vi "readData.vi"(8 "error in (no error)":errorcluster, 10 "Header":T1, 11 "M1M3SAL in":refnum<class "M1M3SAL.lvclass">) -> (0 "error out":errorcluster, 2 "Data":variant, 3 "M1M3SAL out":refnum<class "M1M3SAL.lvclass">)   [LabVIEW 2016, in "M1M3SupportCommunicator.lvlib" / "M1M3SAL.lvclass"]
uses:
  M1M3SAL.lvclass
  DataTypes/MessageHeader.ctl
  DataTypes/MessageTypes.ctl
  DataTypes/MessageTopics.ctl
  Common_RT_Utilities/U8ArrayParserAutoIndexing/U8ArrayParserAutoIndexing.lvclass
  M1M3SupportCommunicator.lvlib
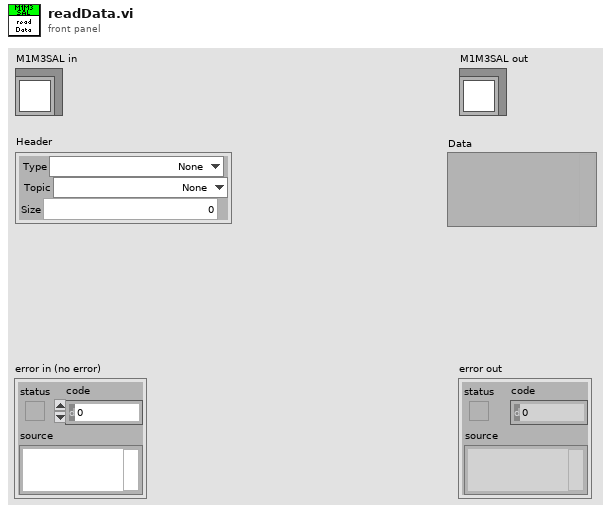
[diagram p1: front panel]
types:
  T1 = typedef "M1M3SupportCommunicator.lvlib/MessageHeader.ctl" = cluster{"Type":T2, "Topic":T3, "Size":i32}
  T2 = typedef "M1M3SupportCommunicator.lvlib/MessageTypes.ctl" = enum8{"None", "PutSample", "GetNextSample", "LogEvent", "GetEvent", "IssueCommand", "CommandId", "WaitForCompletion", "AcceptCommand", "AckCommand"}
  T3 = typedef "M1M3SupportCommunicator.lvlib/MessageTopics.ctl" = enum8{"None", "ForceActuatorData", "MirrorForceData", "HardpointData", "AirData", "DynamicData", "FPGAData", "IMSData", "ForceActuatorStatus", "ElevationData", "HardpointStatus", "HardpointActuatorChase", "AirStatus", "ForceActuatorSafetyChecks", "ForceActuatorTest", "ActuatorBroadcastCounter", "StatusChecks", "CellChecks", "HardpointActuatorBreakaway", "RaiseMirrorComplete", "ILCCommunication", "ElevationAngleChecks", "DetailedState", "ServoLoops", "ForceActuatorInfo", "LowerMirrorComplete", "HardpointActuatorInfo", "SettingsApplied", "ErrorCode", "StartupChecks", "SummaryState", "SettingVersions", "ActuatorTestStatus", "AppliedSettingsMatchStart", "Enable", "EnterMaintenance", "Standby", "AbortLowerM1M3", "ApplyAberrationByForces", "ApplyAOSCorrectionByBendingModes", "ClearAOSCorrection", "Start", "RaiseM1M3", "TestForceActuator", "LowerM1M3", "ApplyAOSCorrectionByForces", "Disable", "ApplyAberationByBendingMode", "TestHardpoint", "ManipulateM1M3", "ClearAberration", "Exit", "TestAir", "AbortRaiseM1M3", "MoveHardpointActuators", "ExitMaintenance", "Shutdown"}
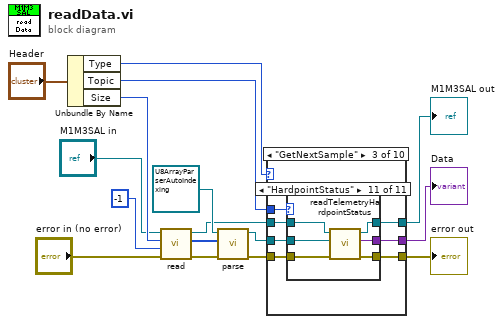
[diagram p0: block diagram]
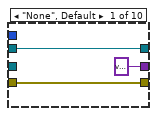
[diagram p2: hidden frame]
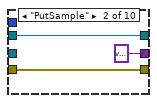
[diagram p3: hidden frame]
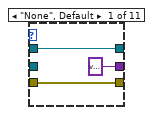
[diagram p4: hidden frame]
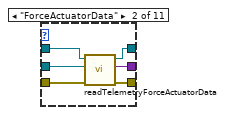
[diagram p5: hidden frame]
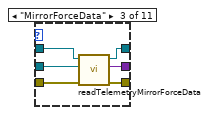
[diagram p6: hidden frame]
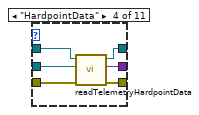
[diagram p7: hidden frame]
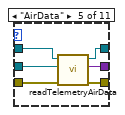
[diagram p8: hidden frame]
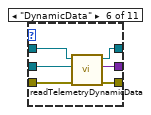
[diagram p9: hidden frame]
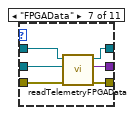
[diagram p10: hidden frame]
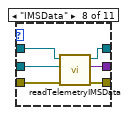
[diagram p11: hidden frame]
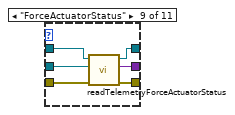
[diagram p12: hidden frame]
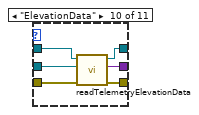
[diagram p13: hidden frame]
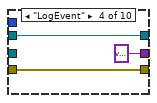
[diagram p14: hidden frame]
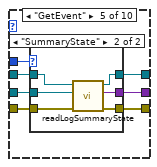
[diagram p15: hidden frame]
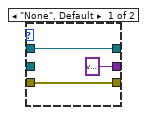
[diagram p16: hidden frame]
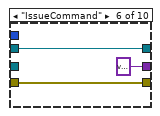
[diagram p17: hidden frame]
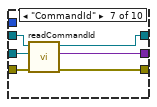
[diagram p18: hidden frame]
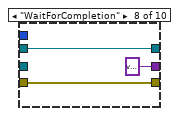
[diagram p19: hidden frame]
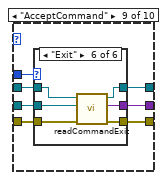
[diagram p20: hidden frame]
diagram:
  n1 = Unbundle By Name("Header") -> ("Type"=w1:T2, "Topic"=w15:T3, "Size"=w14:i32)
  n2 = call "read.vi"("error in (no error)"="error in (no error)", "Timeout"=-1, "NumberOfBytes"=w14, "M1M3SAL in"="M1M3SAL in") -> ("error out"=w6:errorcluster, "Data"=w10:u8[], "M1M3SAL out"=w9:refnum<class "M1M3SAL.lvclass">)  [unwired: 4 in, 1 out]
  n3 = call "parse.vi"("error in (no error)"=w6, "Data"=w10, "U8ArrayParserAutoIndexing in"=refnum<class "U8ArrayParserAutoIndexing.lvclass"> refnum ("RTUtilities.lvlib:U8ArrayParserAutoIndexing.lvclass")) -> ("error out"=w7:errorcluster, "U8ArrayParserAutoIndexing out"=w8:refnum<class "U8ArrayParserAutoIndexing.lvclass">)  [unwired: 7 in]
  n4 = case shown="\"GetNextSample\"" w1 {
    tunnel: w15 -> [_ _ w29 _ w96 _ _ _ w130 _]
    tunnel: w9 -> [w19 w22 w27 w95 w102 w114 w119 w123 w129 w166]
    tunnel: w8 -> [_ _ w23 _ w101 _ w118 _ w128 _]
    tunnel: w7 -> [w17 w21 w25 w93 w100 w113 w117 w121 w127 w164]
    tunnel: [w19 w22 w28 w95 w97 w114 w116 w123 w126 w166] -> w4
    tunnel: [variant ("EventSummaryState") variant ("EventSummaryState") w24 variant ("EventSummaryState") w98 variant ("EventSummaryState") w120 variant ("EventSummaryState") w125 variant ("EventSummaryState")] -> w3
    tunnel: [w17 w21 w26 w93 w99 w113 w115 w121 w124 w164] -> w2
    frame "None", Default {
    }
    frame "PutSample" {
    }
    frame "GetNextSample" {
      n5 = case shown="\"HardpointStatus\"" w29 {
        tunnel: [w32 w33 w43 w49 w55 w61 w67 w73 w79 w85 w91] -> w28
        tunnel: w27 -> [w32 w38 w44 w50 w56 w62 w68 w74 w80 w86 w92]
        tunnel: [w31 w35 w40 w46 w53 w58 w65 w71 w75 w82 w88] -> w26
        tunnel: w25 -> [w31 w36 w41 w47 w52 w59 w64 w70 w77 w83 w89]
        tunnel: [variant ("EventSummaryState") w34 w39 w45 w54 w57 w66 w72 w76 w81 w87] -> w24
        tunnel: w23 -> [_ w37 w42 w48 w51 w60 w63 w69 w78 w84 w90]
        frame "None", Default {
        }
        frame "ForceActuatorData" {
          n6 = call "readTelemetryForceActuatorData.vi"("error in (no error)"=w36, "Parser"=w37, "M1M3SAL in"=w38) -> ("error out"=w35:errorcluster, "EventSummaryState"=w34:variant, "M1M3SAL out"=w33:refnum<class "M1M3SAL.lvclass">)  [unwired: 6 in]
        }
        frame "MirrorForceData" {
          n7 = call "readTelemetryMirrorForceData.vi"("error in (no error)"=w41, "Parser"=w42, "M1M3SAL in"=w44) -> ("error out"=w40:errorcluster, "EventSummaryState"=w39:variant, "M1M3SAL out"=w43:refnum<class "M1M3SAL.lvclass">)  [unwired: 6 in]
        }
        frame "HardpointData" {
          n8 = call "readTelemetryHardpointData.vi"("error in (no error)"=w47, "Parser"=w48, "M1M3SAL in"=w50) -> ("error out"=w46:errorcluster, "EventSummaryState"=w45:variant, "M1M3SAL out"=w49:refnum<class "M1M3SAL.lvclass">)  [unwired: 6 in]
        }
        frame "AirData" {
          n9 = call "readTelemetryAirData.vi"("error in (no error)"=w52, "Parser"=w51, "M1M3SAL in"=w56) -> ("error out"=w53:errorcluster, "EventSummaryState"=w54:variant, "M1M3SAL out"=w55:refnum<class "M1M3SAL.lvclass">)  [unwired: 6 in]
        }
        frame "DynamicData" {
          n10 = call "readTelemetryDynamicData.vi"("error in (no error)"=w59, "Parser"=w60, "M1M3SAL in"=w62) -> ("error out"=w58:errorcluster, "EventSummaryState"=w57:variant, "M1M3SAL out"=w61:refnum<class "M1M3SAL.lvclass">)  [unwired: 6 in]
        }
        frame "FPGAData" {
          n11 = call "readTelemetryFPGAData.vi"("error in (no error)"=w64, "Parser"=w63, "M1M3SAL in"=w68) -> ("error out"=w65:errorcluster, "EventSummaryState"=w66:variant, "M1M3SAL out"=w67:refnum<class "M1M3SAL.lvclass">)  [unwired: 6 in]
        }
        frame "IMSData" {
          n12 = call "readTelemetryIMSData.vi"("error in (no error)"=w70, "Parser"=w69, "M1M3SAL in"=w74) -> ("error out"=w71:errorcluster, "EventSummaryState"=w72:variant, "M1M3SAL out"=w73:refnum<class "M1M3SAL.lvclass">)  [unwired: 6 in]
        }
        frame "ForceActuatorStatus" {
          n13 = call "readTelemetryForceActuatorStatus.vi"("error in (no error)"=w77, "Parser"=w78, "M1M3SAL in"=w80) -> ("error out"=w75:errorcluster, "EventSummaryState"=w76:variant, "M1M3SAL out"=w79:refnum<class "M1M3SAL.lvclass">)  [unwired: 6 in]
        }
        frame "ElevationData" {
          n14 = call "readTelemetryElevationData.vi"("error in (no error)"=w83, "Parser"=w84, "M1M3SAL in"=w86) -> ("error out"=w82:errorcluster, "EventSummaryState"=w81:variant, "M1M3SAL out"=w85:refnum<class "M1M3SAL.lvclass">)  [unwired: 6 in]
        }
        frame "HardpointStatus" {
          n15 = call "readTelemetryHardpointStatus.vi"("error in (no error)"=w89, "Parser"=w90, "M1M3SAL in"=w92) -> ("error out"=w88:errorcluster, "EventSummaryState"=w87:variant, "M1M3SAL out"=w91:refnum<class "M1M3SAL.lvclass">)  [unwired: 6 in]
        }
      }
    }
    frame "LogEvent" {
    }
    frame "GetEvent" {
      n16 = case shown="\"SummaryState\"" w96 {
        tunnel: [variant ("CommandEnterControl") w107] -> w98
        tunnel: [w103 w108] -> w97
        tunnel: [w104 w106] -> w99
        tunnel: w102 -> [w103 w111]
        tunnel: w101 -> [_ w110]
        tunnel: w100 -> [w104 w109]
        frame "None", Default {
        }
        frame "SummaryState" {
          n17 = call "readLogSummaryState.vi"("error in (no error)"=w109, "Parser"=w110, "M1M3SAL in"=w111) -> ("error out"=w106:errorcluster, "EventSummaryState"=w107:variant, "M1M3SAL out"=w108:refnum<class "M1M3SAL.lvclass">)  [unwired: 6 in]
        }
      }
    }
    frame "IssueCommand" {
    }
    frame "CommandId" {
      n18 = call "readCommandId.vi"("error in (no error)"=w117, "Parser"=w118, "M1M3SAL in"=w119) -> ("error out"=w115:errorcluster, "CommandId"=w120:variant, "M1M3SAL out"=w116:refnum<class "M1M3SAL.lvclass">)  [unwired: 6 in]
    }
    frame "WaitForCompletion" {
    }
    frame "AcceptCommand" {
      n19 = case shown="\"Exit\"" w130 {
        tunnel: [variant ("CommandEnterControl") w135 w141 w147 w153 w159] -> w125
        tunnel: [w131 w136 w142 w148 w154 w160] -> w126
        tunnel: [w132 w134 w140 w146 w152 w158] -> w124
        tunnel: w129 -> [w131 w139 w145 w151 w157 w163]
        tunnel: w128 -> [_ w138 w144 w150 w156 w162]
        tunnel: w127 -> [w132 w137 w143 w149 w155 w161]
        frame "None", Default {
        }
        frame "Start" {
          n20 = call "readCommandStart.vi"("error in (no error)"=w137, "Parser"=w138, "M1M3SAL in"=w139) -> ("error out"=w134:errorcluster, "CommandStart"=w135:variant, "M1M3SAL out"=w136:refnum<class "M1M3SAL.lvclass">)  [unwired: 6 in]
        }
        frame "MirrorForceData" {
          n21 = call "readCommandEnable.vi"("error in (no error)"=w143, "Parser"=w144, "M1M3SAL in"=w145) -> ("error out"=w140:errorcluster, "CommandEnable"=w141:variant, "M1M3SAL out"=w142:refnum<class "M1M3SAL.lvclass">)  [unwired: 6 in]
        }
        frame "Disable" {
          n22 = call "readCommandDisable.vi"("error in (no error)"=w149, "Parser"=w150, "M1M3SAL in"=w151) -> ("error out"=w146:errorcluster, "CommandDisable"=w147:variant, "M1M3SAL out"=w148:refnum<class "M1M3SAL.lvclass">)  [unwired: 6 in]
        }
        frame "Standby" {
          n23 = call "readCommandStandby.vi"("error in (no error)"=w155, "Parser"=w156, "M1M3SAL in"=w157) -> ("error out"=w152:errorcluster, "CommandStandby"=w153:variant, "M1M3SAL out"=w154:refnum<class "M1M3SAL.lvclass">)  [unwired: 6 in]
        }
        frame "Exit" {
          n24 = call "readCommandExit.vi"("error in (no error)"=w161, "Parser"=w162, "M1M3SAL in"=w163) -> ("error out"=w158:errorcluster, "CommandExit"=w159:variant, "M1M3SAL out"=w160:refnum<class "M1M3SAL.lvclass">)  [unwired: 6 in]
        }
      }
    }
    frame "AckCommand" {
    }
  }
  "error out" <- w2
  "M1M3SAL out" <- w4
  "Data" <- w3
